vi "Stimulus-Is Active Rep.vi"(0 "Advanced.Rep Mask":string, 9 "Rep Num":i32, 11 "error in (no error)":errorcluster) -> (8 "Is Active":bool, 10 "Multiplier":dbl, 15 "error out":errorcluster)   [LabVIEW 2020]
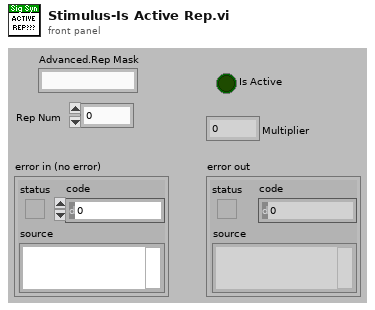
[diagram p1: front panel]
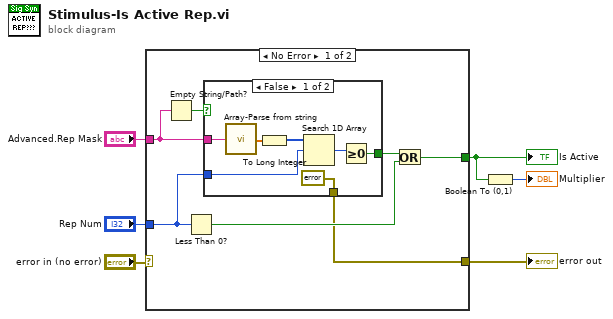
[diagram p0: block diagram]
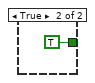
[diagram p2: hidden frame]
diagram:
  n1 = case shown="No Error" "error in (no error)" {
    selector: "error in (no error)" -> [_ w22]
    tunnel: [w7 w22] -> w5
    tunnel: "Advanced.Rep Mask" -> [w13 _]
    tunnel: "Rep Num" -> [w10 _]
    tunnel: [w8 _] -> w2
    frame No Error {
      n2 = Empty String/Path?(string/path=w13) -> (empty?=w12:bool)
      n3 = Less Than 0?(x=w10) -> (x < 0?=w9:bool)
      n4 = case shown="False" w12 {
        tunnel: w13 -> [w20 _]
        tunnel: w10 -> [w17 _]
        tunnel: [w15 TRUE] -> w11
        tunnel: [errorcluster {"status"=TRUE, "code"=0, "source"="This use of advanced tab is deprecated!"} ("error IO") _] -> w7
        frame False {
          n5 = call "Array-Parse from string.vi"("String"=w20) -> ("Array"=w19:dbl[])  [unwired: 13 in, 1 out]
          n6 = To Long Integer(number=w19) -> (32bit integer=w18:i32[])
          n7 = Search 1D Array(1D array=w18, element=w17) -> (index of element=w16:i32)  [unwired: 1 in]
          n8 = Greater Or Equal To 0?(x=w16) -> (x >= 0?=w15:bool)
        }
        frame True {
        }
      }
      n9 = Or(x=w11, y=w9) -> (x .or. y?=w8:bool)
    }
    frame Error {
    }
  }
  "error out" <- w5
  "Is Active" <- w2
  n10 = Boolean To (0,1)(Boolean=w2) -> (0, 1=→"Multiplier":i16)
